vi "CRYChange Limits Flatten Data by One.vi"(7 "Option":string, 10 "Value":dbl format="%.2f", 11 "Flatten Limits In":string) -> (0 "Error?":bool, 3 "Flatten Limits Out":string)   [LabVIEW 2013]
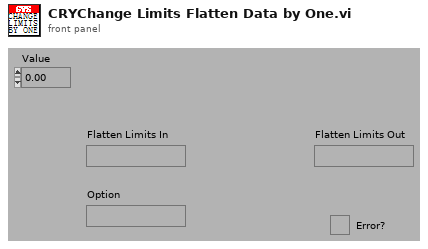
[diagram p1: front panel]
types:
  T1 = typedef "CRYLimits.ctl" = cluster{"Name":string, "Tolerance":u16, "X Axis":u16, "Limits":u16, "Upper Limit":cluster{dbl, dbl}[], "Align Ref":cluster{dbl, dbl}, "Lower Limit":cluster{dbl, dbl}[], "Y data":u16, "Y unit":string, "Y dB ref":dbl, "Curve Names":string[], "Y-Resolution":u8, "Type":u16, "x float":bool, "X min-max-step":cluster{"Limit X Offset Min":dbl, "Limit X Offset Max":dbl, "Limit X Offset Step Size":dbl}, "magn/phase":u16, "Upper Limit Type":u16, "Lower Limit Type":u16, "Lim Curve axis up":u16, "Lim Curve axis lo":u16, "Data Selection Upper":u16, "Data Selection Lower":u16, "X-Resolution":u8, "Output failed point curves?":bool, "X data":u16, "X unit":string, "X dB ref":dbl, "X-Y Graph Set-up":string, "Tab Value":enum32{"Data", "Parameters"}, "Help":string, "X Up Val":dbl, "Y Up Val":dbl, "X Low Val":dbl, "Y Low Val":dbl, "Up Limit Val":dbl, "Low Limit Val":dbl, "bAdd DataName":bool, "Custom Name":string}
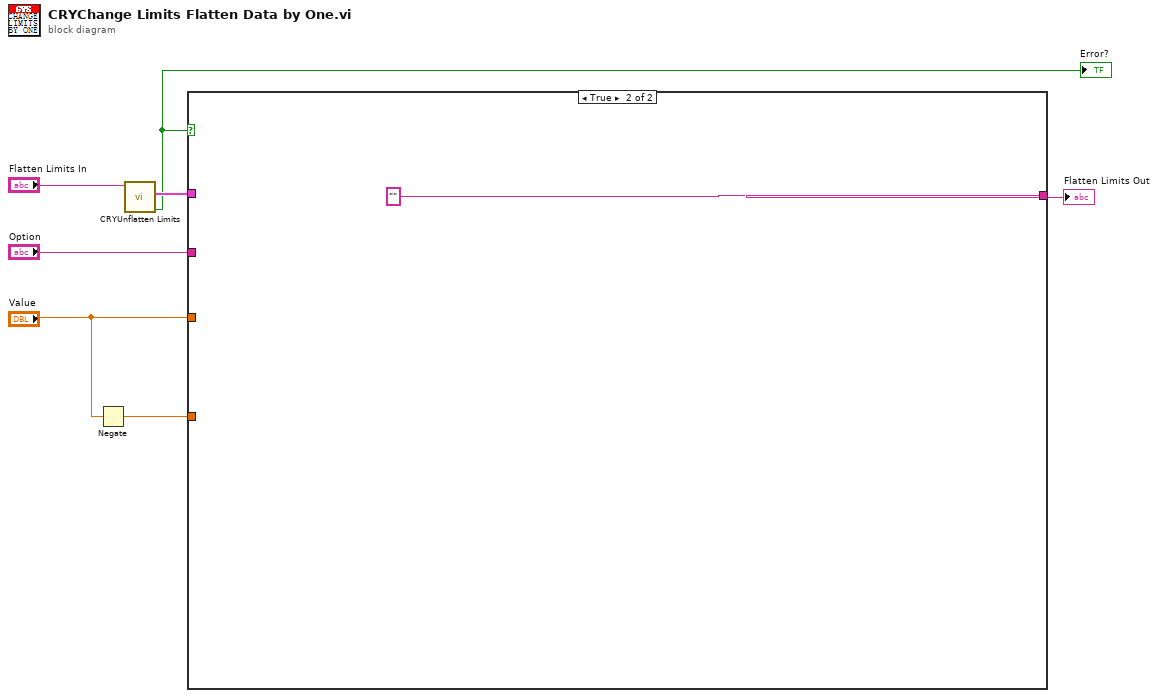
[diagram p0: block diagram]
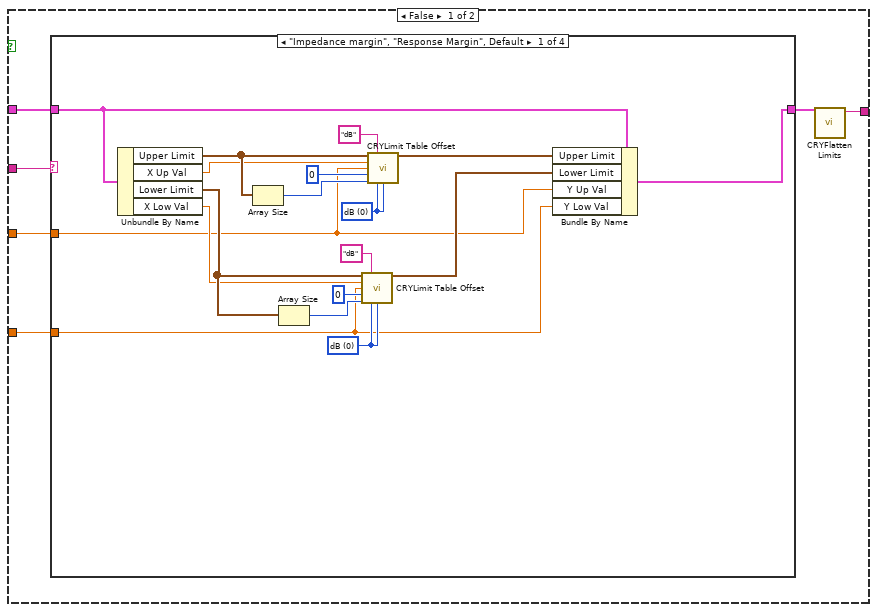
[diagram p2: hidden frame]
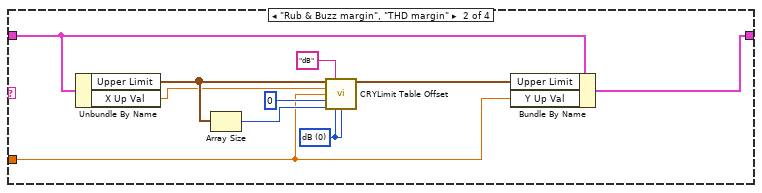
[diagram p3: hidden frame]
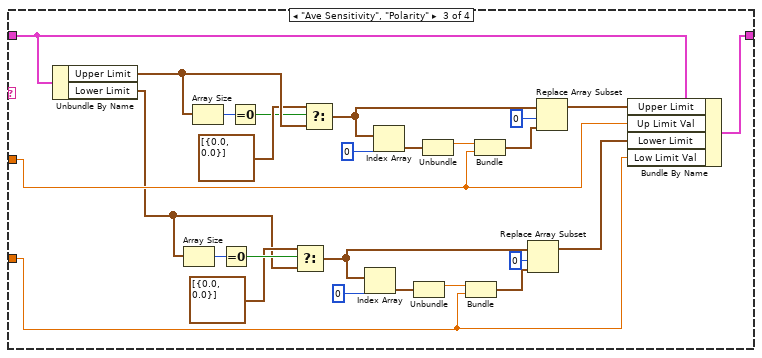
[diagram p4: hidden frame]
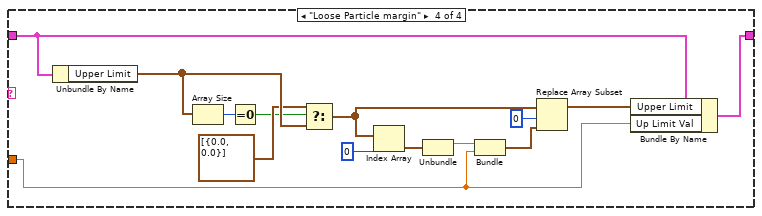
[diagram p5: hidden frame]
diagram:
  n1 = Negate(x="Value") -> (-x=w1:dbl)
  n2 = call "CRYUnflatten Limits.vi"("Unflatten Limits"="Flatten Limits In") -> ("Error?"=w4:bool, "Limits"=w5:T1)  [unwired: 8 in, 1 out]
  "Error?" <- w4
  n3 = case shown="True" w4 {
    tunnel: [w13 "" ("Flatten Limits String")] -> w6
    tunnel: w5 -> [w12 _]
    tunnel: "Option" -> [w10 _]
    tunnel: "Value" -> [w9 _]
    tunnel: w1 -> [w8 _]
    frame False {
      n4 = case shown="\"Impedance margin\", \"Response Margin\", Default" w10 {
        tunnel: w12 -> [w22 w36 w55 w69]
        tunnel: [w21 w35 w56 w70] -> w11
        tunnel: w9 -> [w15 w32 w45 w68]
        tunnel: w8 -> [w14 _ w43 _]
        frame "Impedance margin", "Response Margin", Default {
          w24 = u16 0 items=["dB", "%"] ("x Unit")
          w30 = u16 0 items=["dB", "%"] ("x Unit")
          n5 = Unbundle By Name(w22) -> ("Upper Limit"=w28:cluster{dbl, dbl}[], "X Up Val"=w18:dbl, "Lower Limit"=w17:cluster{dbl, dbl}[], "X Low Val"=w16:dbl)
          n6 = Array Size(array=w28) -> (size(s)=w27:i32)
          n7 = Array Size(array=w17) -> (size(s)=w26:i32)
          n8 = call "CRYLimit Table Offset.vi"("Limit in"=w17, "Data unit"="dB", "X offset"=w16, "Y offset"=w14, "Starting Column"=0, "Number of columns"=w26, "x Unit"=w24, "y Unit"=w24) -> ("Limit out"=w19:cluster{"Numeric":dbl, "Log Out":dbl}[])  [unwired: 2 in, 5 out]
          n9 = call "CRYLimit Table Offset.vi"("Limit in"=w28, "Data unit"="dB", "X offset"=w18, "Y offset"=w15, "Starting Column"=0, "Number of columns"=w27, "x Unit"=w30, "y Unit"=w30) -> ("Limit out"=w20:cluster{"Numeric":dbl, "Log Out":dbl}[])  [unwired: 2 in, 5 out]
          n10 = Bundle By Name(cluster=w22, "Upper Limit"=w20, "Lower Limit"=w19, "Y Up Val"=w15, "Y Low Val"=w14) -> (w21:T1)
        }
        frame "Rub & Buzz margin", "THD margin" {
          w40 = u16 0 items=["dB", "%"] ("x Unit")
          n11 = Unbundle By Name(w36) -> ("Upper Limit"=w38:cluster{dbl, dbl}[], "X Up Val"=w33:dbl)
          n12 = Array Size(array=w38) -> (size(s)=w37:i32)
          n13 = call "CRYLimit Table Offset.vi"("Limit in"=w38, "Data unit"="dB", "X offset"=w33, "Y offset"=w32, "Starting Column"=0, "Number of columns"=w37, "x Unit"=w40, "y Unit"=w40) -> ("Limit out"=w34:cluster{"Numeric":dbl, "Log Out":dbl}[])  [unwired: 2 in, 5 out]
          n14 = Bundle By Name(cluster=w36, "Upper Limit"=w34, "Y Up Val"=w32) -> (w35:T1)
        }
        frame "Ave Sensitivity", "Polarity" {
          n15 = Unbundle By Name(w55) -> ("Upper Limit"=w66:cluster{dbl, dbl}[], "Lower Limit"=w44:cluster{dbl, dbl}[])
          n16 = Array Size(array=w44) -> (size(s)=w49:i32)
          n17 = Array Size(array=w66) -> (size(s)=w63:i32)
          n18 = Equal To 0?(x=w49) -> (x = 0?=w48:bool)
          n19 = Equal To 0?(x=w63) -> (x = 0?=w64:bool)
          n20 = Select(t=cluster{dbl, dbl}[] [{0.0, 0.0}] ("Upper Limit"), s=w48, f=w44) -> (s? t:f=w46:cluster{dbl, dbl}[])
          n21 = Select(t=cluster{dbl, dbl}[] [{0.0, 0.0}] ("Upper Limit"), s=w64, f=w66) -> (s? t:f=w67:cluster{dbl, dbl}[])
          n22 = Index Array(array=w46, index=0) -> (element=w51:cluster{dbl, dbl})
          n23 = Index Array(array=w67, index=0) -> (element=w60:cluster{dbl, dbl})
          n24 = Unbundle(w51) -> (w52:dbl)  [unwired: 1 out]
          n25 = Unbundle(w60) -> (w59:dbl)  [unwired: 1 out]
          n26 = Bundle(w52, w43) -> (w53:cluster{dbl, dbl})  [unwired: 1 out]
          n27 = Bundle(w59, "Value"=w45) -> (w58:cluster{dbl, "Value":dbl})  [unwired: 1 out]
          n28 = Replace Array Subset(array=w46, new element=w53, index=0) -> (w42:cluster{dbl, dbl}[])
          n29 = Replace Array Subset(array=w67, new element=w58, index=0) -> (w62:cluster{dbl, dbl}[])
          n30 = Bundle By Name(cluster=w55, "Upper Limit"=w62, "Up Limit Val"=w45, "Lower Limit"=w42, "Low Limit Val"=w43) -> (w56:T1)
        }
        frame "Loose Particle margin" {
          n31 = Unbundle By Name(w69) -> ("Upper Limit"=w80:cluster{dbl, dbl}[])
          n32 = Array Size(array=w80) -> (size(s)=w77:i32)
          n33 = Equal To 0?(x=w77) -> (x = 0?=w78:bool)
          n34 = Select(t=cluster{dbl, dbl}[] [{0.0, 0.0}] ("Upper Limit"), s=w78, f=w80) -> (s? t:f=w81:cluster{dbl, dbl}[])
          n35 = Index Array(array=w81, index=0) -> (element=w74:cluster{dbl, dbl})
          n36 = Unbundle(w74) -> (w73:dbl)  [unwired: 1 out]
          n37 = Bundle(w73, "Value"=w68) -> (w72:cluster{dbl, "Value":dbl})  [unwired: 1 out]
          n38 = Replace Array Subset(array=w81, new element=w72, index=0) -> (w76:cluster{dbl, dbl}[])
          n39 = Bundle By Name(cluster=w69, "Upper Limit"=w76, "Up Limit Val"=w68) -> (w70:T1)
        }
      }
      n40 = call "CRYFlatten Limits.vi"("Limits"=w11) -> ("Flatten Limits String"=w13:string)  [unwired: 10 in]
    }
    frame True {
    }
  }
  "Flatten Limits Out" <- w6
